vi "Increment.vi"(6 "Labels":map{string, string}(c390), 8 "error in (no error)":errorcluster, 10 "Step":dbl=1.0, 11 "Gauge Ref":refnum<data-value>) -> (0 "error out":errorcluster, 3 "Gauge Ref out":refnum<data-value>)   [LabVIEW 2020, in "Metrics.lvlib" / "Gauge.lvclass"]
doc: "Increments the value of the gauge metric."
uses:
  Gauge.lvclass
  C:/Github-locals/PromVIEW/src/metrics/metric/Metric.lvclass
  metric/Metric.lvclass/Metric.ctl
  sample/Sample.lvclass/Sample.ctl
  metric/Read Samples.vi
  sample/Read Value.vi
  sample/Write Value.vi
  sample/Write Labels.vi
  metric/Write Samples.vi
  sample/Sample.lvclass
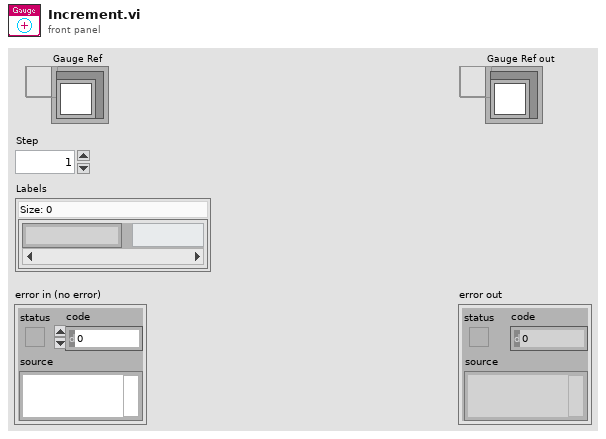
[diagram p1: front panel]
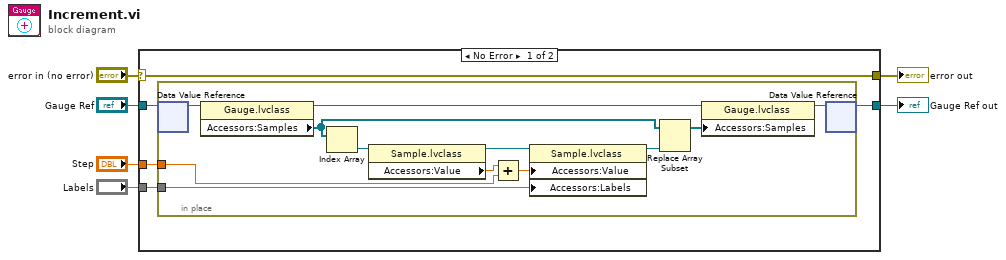
[diagram p0: block diagram]
diagram:
  n1 = case shown="No Error" "error in (no error)" {
    selector: "error in (no error)" -> [w11 w24]
    tunnel: [w11 w24] -> w5
    tunnel: "Gauge Ref" -> [w10 _]
    tunnel: "Step" -> [w9 _]
    tunnel: "Labels" -> [w8 _]
    tunnel: [w7 _] -> w1
    frame No Error {
      n2 = in-place {
        in-place-border: w9 -> [w14]
        in-place-border: w8 -> [w12]
        n3 = in-place-dvr #1(w10) -> (w23:refnum<class "Gauge.lvclass">)  [unwired: 1 out]
        n4 = property class="Gauge.lvclass"(reference=w23) -> (reference out=w17:refnum<class "Gauge.lvclass">, "Accessors:Samples"=w20:refnum<class "Sample.lvclass">[])  [unwired: 1 in, 1 out]
        n5 = Index Array(array=w20) -> (element=w22:refnum<class "Sample.lvclass">)  [unwired: 1 in]
        n6 = property class="Sample.lvclass"(reference=w22) -> (reference out=w21:refnum<class "Sample.lvclass">, "Accessors:Value"=w15:dbl)  [unwired: 1 in, 1 out]
        n7 = Add(x=w15, y=w14) -> (x+y=w13:dbl)
        n8 = property class="Sample.lvclass"(reference=w21, "Accessors:Value"=w13, "Accessors:Labels"=w12) -> (reference out=w19:refnum<class "Sample.lvclass">)  [unwired: 1 in, 1 out]
        n9 = Replace Array Subset(array=w20, new element=w19) -> (w18:refnum<class "Sample.lvclass">[])  [unwired: 1 in]
        n10 = property class="Gauge.lvclass"(reference=w17, "Accessors:Samples"=w18) -> (reference out=w16:refnum<class "Gauge.lvclass">)  [unwired: 1 in, 1 out]
        n11 = in-place-dvr #1(w16) -> (w7:refnum<data-value>)  [unwired: 1 out]
      }
    }
    frame Error {
    }
  }
  "error out" <- w5
  "Gauge Ref out" <- w1
